vi "CheckCreateFile.vi"(8 "Error In":errorcluster, 10 "Folder":string, 11 "Image Name":string) -> (0 "Error Out":errorcluster, 3 "File Path":path)   [LabVIEW 2013]
doc: "VI Checks for a folder in the application\ndirectory. If it doesn't existe, the VI\ncreates the folder and returns the path of the\nimage that is being saved there. \n\nAlso checks to see if image already exists. If so, increments\nthe last number character before .jpg and saves the new image\nin the directory above."
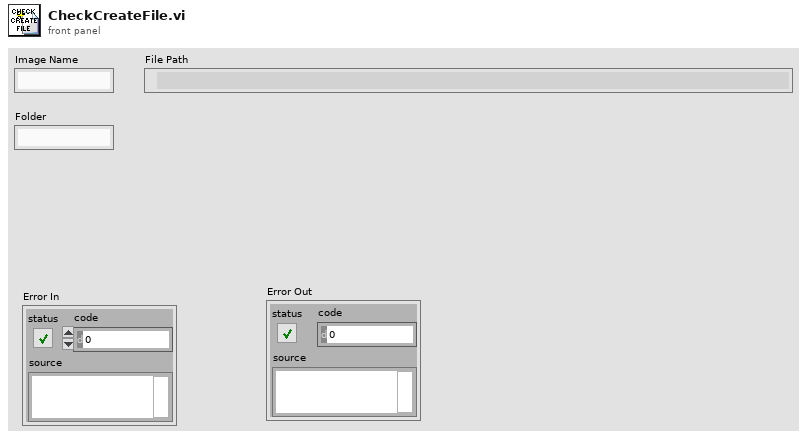
[diagram p1: front panel]
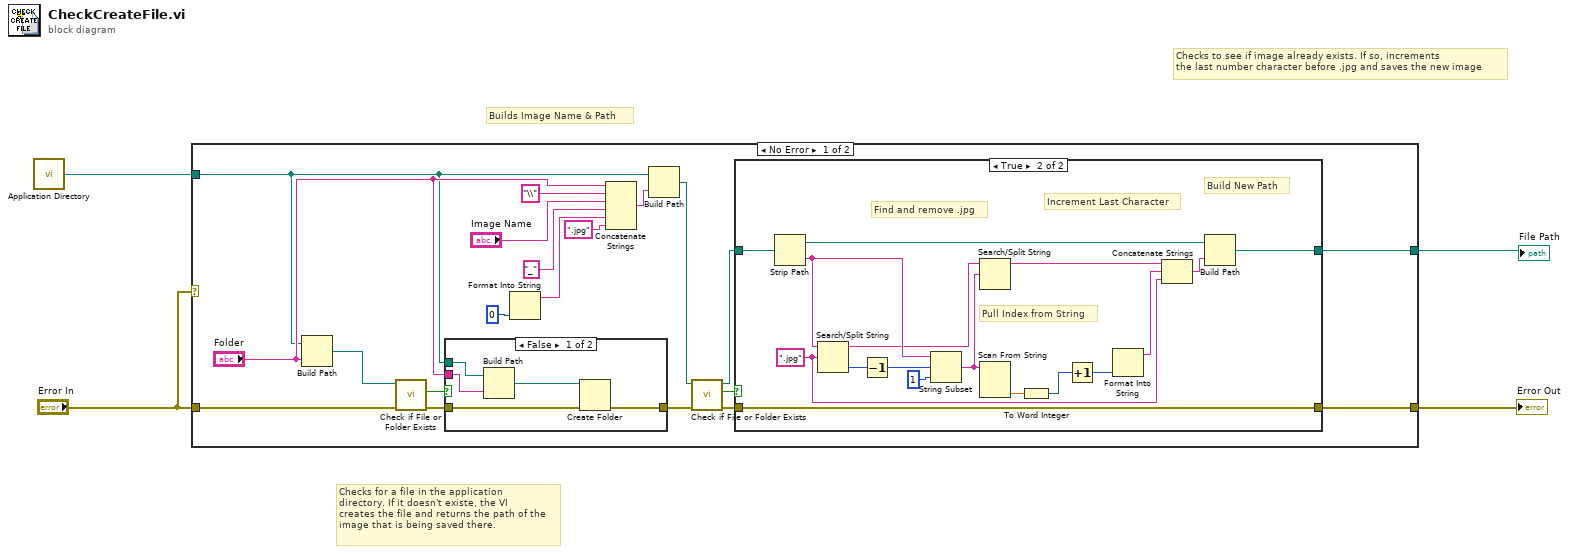
[diagram p0: block diagram]
diagram:
  # "Builds Image Name & Path"
  # "Checks to see if image already exists. If so, increments\nthe last number character before .jpg and saves the new image"
  # "Checks for a file in the application\ndirectory. If it doesn't existe, the VI\ncreates the file and returns the path of the\nimage that is being saved there."
  n1 = call <vilib>:"Application Directory.vi"() -> ("Application Directory"=w1:path)
  n2 = case shown="No Error" "Error In" {
    tunnel: "Error In" -> [w9 w51]
    tunnel: [w8 w51] -> w4
    tunnel: [w6 w50] -> w2
    tunnel: w1 -> [w5 w50]
    frame No Error {
      n3 = Build Path(base path=w5, name or relative path="Folder") -> (appended path=w23:path)
      n4 = call <vilib>:"Check if File or Folder Exists.vi"("error in (no error)"=w9, "path"=w23) -> ("error out"=w24:errorcluster, "file or folder exists?"=w22:bool)  [unwired: 7 in, 1 out]
      n5 = case shown="False" w22 {
        tunnel: w5 -> [w48 _]
        tunnel: "Folder" -> [w46 _]
        tunnel: [w45 w49] -> w10
        tunnel: w24 -> [w44 w49]
        frame False {
          n6 = Build Path(base path=w48, name or relative path=w46) -> (appended path=w47:path)
          n7 = Create Folder(path (use dialog)=w47, error in=w44) -> (error out=w45:errorcluster)  [unwired: 1 in, 2 out]
        }
        frame True {
        }
      }
      n8 = Format Into String(0) -> (resulting string=w14:string)  [unwired: 3 in, 1 out]
      n9 = Concatenate Strings("Folder", "\\" ("string"), "Image Name", "_" ("string"), w14, ".jpg" ("string")) -> (w19:string)
      n10 = Build Path(base path=w5, name or relative path=w19) -> (appended path=w13:path)
      n11 = call <vilib>:"Check if File or Folder Exists.vi"("error in (no error)"=w10, "path"=w13) -> ("error out"=w7:errorcluster, "file or folder exists?"=w12:bool, "dup path"=w11:path)  [unwired: 7 in]
      n12 = case shown="True" w12 {
        tunnel: w11 -> [w26 w43]
        tunnel: [w26 w30] -> w6
        tunnel: [w25 w27] -> w8
        tunnel: w7 -> [w25 w27]
        frame False {
        }
        frame True {
          w32 = ".jpg" ("search string/char (-)")
          # "Build New Path"
          # "Increment Last Character"
          # "Find and remove .jpg"
          # "Pull Index from String"
          n13 = Strip Path(path=w43) -> (stripped path=w33:path, name=w42:string)
          n14 = Search/Split String(string=w42, search string/char (-)=w32) -> (substring before match=w37:string, offset of match=w40:i32)  [unwired: 1 in, 1 out]
          n15 = Decrement(x=w40) -> (x-1=w39:i32)
          n16 = String Subset(string=w42, offset (0)=w39, length (rest)=1 ("length (rest)")) -> (substring=w36:string)
          n17 = Search/Split String(string=w37, search string/char (-)=w36) -> (substring before match=w35:string)  [unwired: 1 in, 2 out]
          n18 = Scan From String(input string=w36) -> (output 1=w38:dbl)  [unwired: 4 in, 3 out]
          n19 = To Word Integer(number=w38) -> (16bit integer=w29:i16)
          n20 = Increment(x=w29) -> (x+1=w28:i16)
          n21 = Format Into String(w28) -> (resulting string=w34:string)  [unwired: 3 in, 1 out]
          n22 = Concatenate Strings(w35, w34, w32) -> (w31:string)
          n23 = Build Path(base path=w33, name or relative path=w31) -> (appended path=w30:path)
        }
      }
    }
    frame Error {
    }
  }
  "Error Out" <- w4
  "File Path" <- w2
